vi "GT Set Pt Memory.vi"(8 "error in (no error)":errorcluster caption="错误输入（无错误）", 9 "memory":i16, 10 "profile":i16, 11 "cardNum":i16) -> (0 "error out":errorcluster caption="错误输出", 3 "function return":i16)   [LabVIEW 2014, in "gts.lvlib"]
doc: "GT_API GT_SetPtMemory(short cardNum,short profile,short memory);"
uses:
  gts.lvlib
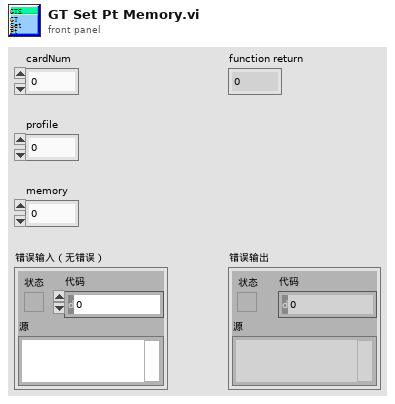
[diagram p1: front panel]
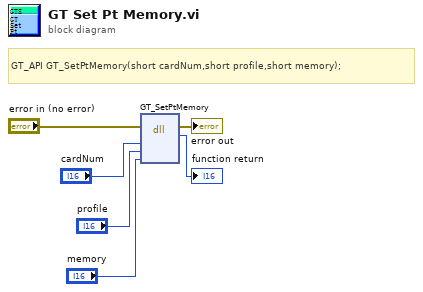
[diagram p0: block diagram]
diagram:
  # "GT_API GT_SetPtMemory(short cardNum,short profile,short memory);"
  n1 = dll-call lib="PTH2habs D固高科技资料GTS控制卡GTS卡18年上半年资料dllVC32bit\nmulti_cardgts.*" fn="GT_SetPtMemory"(error in="error in (no error)", "cardNum"="cardNum", "profile"="profile", "memory"="memory") -> (error out=→"error out":errorcluster, →"function return":i16)  [unwired: 5 in, 1 out]
